vi "S2C_OM8257_Poly_GND.vi"(8 "Error In":errorcluster, 10 "GND":T1={"Current (A)"=1240.0, "Voltage (V)"=10.0, "Hi-Limit (mohm)"=100, "Lo-Limit (mhom)"=0, "Dwell (s)"=1.0, "Offset (mhom)"=0, "Auto Offset"=FALSE, "Frequency (Hz)"=60, "DualCHEK"=0, "Scanner Selection"=0, "Scanner?"=FALSE, "Step Selection"=1, "Add Step"=FALSE} {"DualCHEK" items=["OFF", "ACW", "DCW"]}, 11 "Settings":T2={"Driver"="Omnia8257", "Command"="CfgStep GND", "Return"="ErrorStatus", "Parameters"="", "Timeout"=10.0}) -> (0 "Error Out":errorcluster, 3 "Response":string)   [LabVIEW 2015]
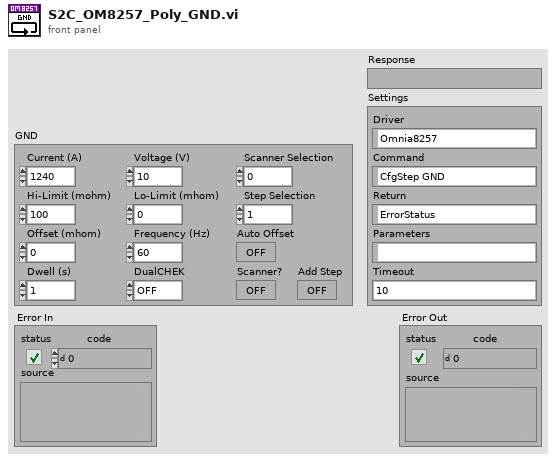
[diagram p1: front panel]
types:
  T1 = cluster{"Current (A)":dbl, "Voltage (V)":dbl, "Hi-Limit (mohm)":u16, "Lo-Limit (mhom)":u16, "Dwell (s)":dbl, "Offset (mhom)":u16, "Auto Offset":bool, "Frequency (Hz)":u16, "DualCHEK":u16, "Scanner Selection":i32, "Scanner?":bool, "Step Selection":i32, "Add Step":bool}
  T2 = cluster{"Driver":string, "Command":string, "Return":string, "Parameters":string, "Timeout":dbl}
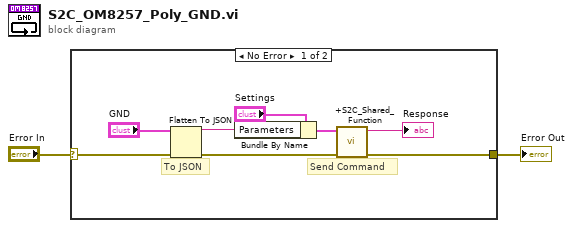
[diagram p0: block diagram]
diagram:
  n1 = case shown="No Error" "Error In" {
    selector: "Error In" -> [w6 w11]
    tunnel: [w5 w11] -> w1
    frame No Error {
      # "To JSON"
      # "Send Command"
      n2 = Flatten To JSON(anything="GND", error in (no error)=w6) -> (JSON string=w7:string, 11:w9:errorcluster)  [unwired: 1 in]
      n3 = Bundle By Name(cluster="Settings", "Parameters"=w7) -> (w10:T2)
      n4 = call "+S2C_Shared_Function.vi"("Error In"=w9, "Settings"=w10) -> ("Error Out"=w5:errorcluster, "Response"=→"Response":string)  [unwired: 8 in]
    }
    frame Error {
    }
  }
  "Error Out" <- w1
